vi "TestTPullse.vi"() -> ()   [LabVIEW 2022 SP3]
panel:
  out "Elapsed Time Text":string
  out "output":bool
  in  "Reset":bool
  in  "trigger":bool
  in  "stop":bool
  in  "TPulse":i32
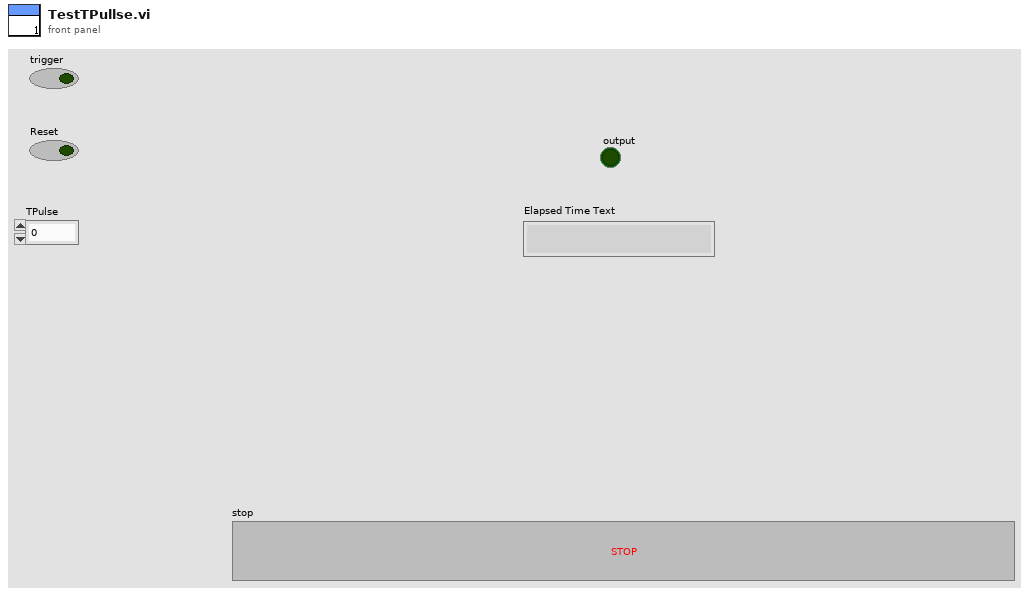
[diagram p1: front panel]
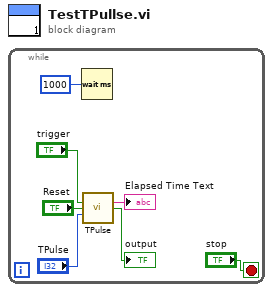
[diagram p0: block diagram]
diagram:
  n1 = while {
    stop <- "stop" stop-if-true
    n2 = Wait (ms)(milliseconds to wait=u32 1000) -> ()  [unwired: 1 out]
    n3 = call "TPulse.vi"("trigger"="trigger", "Reset"="Reset", "TPulse"="TPulse") -> ("Elapsed Time Text"=→"Elapsed Time Text":string, "output"=→"output":bool)  [unwired: 10 in, 1 out]
  }
